vi "Close Continuous Mode.vi"(8 "error in":errorcluster) -> (0 "error out":errorcluster)   [LabVIEW 2017, in "DTACQ - Network Enabled Device Driver.lvlib"]
doc: "Closes the TCP connection and shared variable connections.\n\nNote that the continuous capture mode is different from the other modes, in that a TCP connection remains open the entire time that the driver is running. \n\nExecuting this close method, while the driver is running, will cause an error. This will stop the infinite loop, started by the 'capture continuously' VI."
uses:
  DTACQ - Network Enabled Device Driver.lvlib
  FGV Operaions--Enum.ctl
  Communications/Communications Library.lvlib
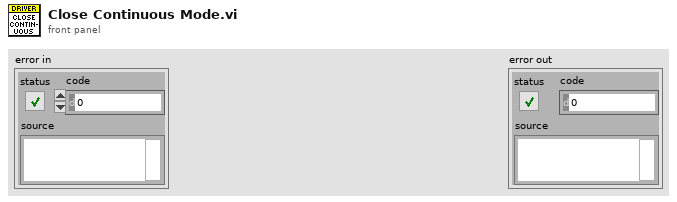
[diagram p1: front panel]
types:
  T1 = typedef "DTACQ - Network Enabled Device Driver.lvlib/FGV Operaions--Enum.ctl" = enum16{"Get Driver Settings", "Set Driver Settings", "Search Variable Names", "Close Connections", "Open Connections", "Get Variable References", "Set Variable References", "Clear"}
  T2 = typedef "DTACQ - Network Enabled Device Driver.lvlib/Driver Global Settings--Typedef.ctl" = cluster{"Waveform Length":i32, "Data Size":T3, "DTACQ Connection Data":T4}
  T3 = typedef "Communications Library.lvlib/Data Size--Enum.ctl" = enum16{"16 Bit (Signed Short)", "32 Bit (Signed Long)"}
  T4 = typedef "Communications Library.lvlib/DTACQ Connection Data--Cluster.ctl" = cluster{"Description":string, "Address":string, "Port":u16, "timeout (ms)":i32, "Termination Character":string, "TCP Connection Reference":refnum<k5>, "Open Connection":bool}
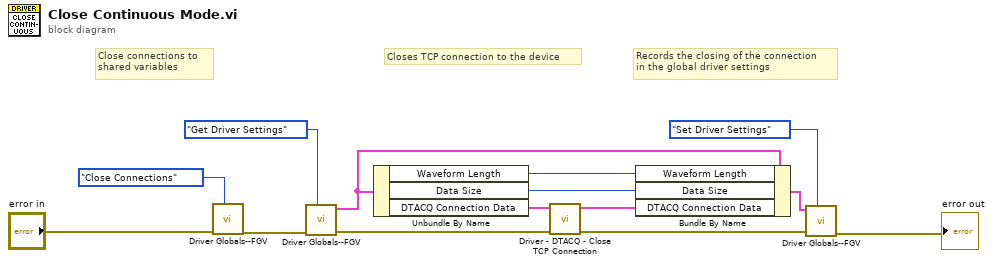
[diagram p0: block diagram]
diagram:
  # "Close connections to \nshared variables"
  # "Records the closing of the connection\nin the global driver settings"
  # "Closes TCP connection to the device"
  n1 = call "Driver Globals--FGV.vi"(7:FGV_Operaions--Enum."Close Connections", "error in"="error in") -> ("error out"=w13:errorcluster)  [unwired: 6 in, 3 out]
  n2 = call "Driver Globals--FGV.vi"(7:FGV_Operaions--Enum."Get Driver Settings", "error in"=w13) -> ("error out"=w10:errorcluster, "Driver Settings Out"=w6:T2)  [unwired: 6 in, 2 out]
  n3 = Unbundle By Name(w6) -> ("Waveform Length"=w4:i32, "Data Size"=w5:T3, "DTACQ Connection Data"=w11:T4)
  n4 = call "Driver - DTACQ - Close TCP Connection.vi"("error in"=w10, "DTACQ Connection Data In"=w11) -> ("error out"=w8:errorcluster, "DTACQ Connection Data Out"=w3:T4)  [unwired: 8 in]
  n5 = Bundle By Name(cluster=w6, "Waveform Length"=w4, "Data Size"=w5, "DTACQ Connection Data"=w3) -> (w2:T2)
  n6 = call "Driver Globals--FGV.vi"(7:FGV_Operaions--Enum."Set Driver Settings", "error in"=w8, "Driver Settings In"=w2) -> ("error out"=→"error out":errorcluster)  [unwired: 5 in, 3 out]
